vi "StopConnection.vi"(8 "ErrorIn":errorcluster, 11 "Reference":T1) -> (0 "ErrorOut":errorcluster)   [LabVIEW 2022 SP3]
uses:
  C:/Users/Robots/Documents/robocadSimLV/assemblies/LibraryForLabVIEW.dll
  assemblies/LibraryForLabVIEW.dll
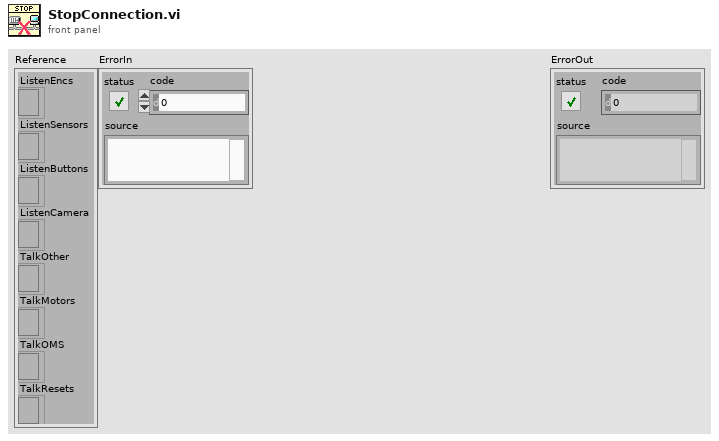
[diagram p1: front panel]
types:
  T1 = cluster{"ListenEncs":refnum<k24>, "ListenSensors":refnum<k24>, "ListenButtons":refnum<k24>, "ListenCamera":refnum<k24>, "TalkOther":refnum<k24>, "TalkMotors":refnum<k24>, "TalkOMS":refnum<k24>, "TalkResets":refnum<k24>}
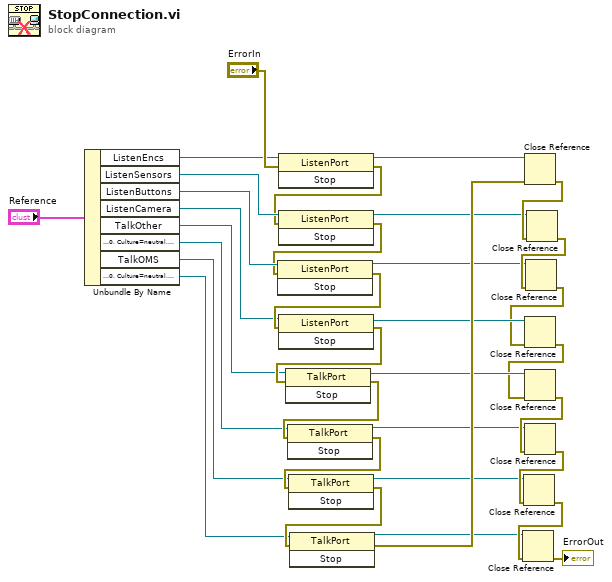
[diagram p0: block diagram]
diagram:
  n1 = Unbundle By Name("Reference") -> ("ListenEncs"=w32:refnum<k24>, "ListenSensors"=w31:refnum<k24>, "ListenButtons"=w29:refnum<k24>, "ListenCamera"=w26:refnum<k24>, "TalkOther"=w24:refnum<k24>, "TalkMotors"=w22:refnum<k24>, "TalkOMS"=w20:refnum<k24>, "TalkResets"=w18:refnum<k24>)
  n2 = invoke class="ListenPort" method="Stop"(reference=w32, error in="ErrorIn") -> (reference out=w17:refnum<k24>, error out=w30:errorcluster)  [unwired: 1 in, 1 out]
  n3 = invoke class="ListenPort" method="Stop"(reference=w31, error in=w30) -> (reference out=w14:refnum<k24>, error out=w28:errorcluster)  [unwired: 1 in, 1 out]
  n4 = invoke class="ListenPort" method="Stop"(reference=w29, error in=w28) -> (reference out=w12:refnum<k24>, error out=w27:errorcluster)  [unwired: 1 in, 1 out]
  n5 = invoke class="ListenPort" method="Stop"(reference=w26, error in=w27) -> (reference out=w11:refnum<k24>, error out=w25:errorcluster)  [unwired: 1 in, 1 out]
  n6 = invoke class="TalkPort" method="Stop"(reference=w24, error in=w25) -> (reference out=w9:refnum<k24>, error out=w23:errorcluster)  [unwired: 1 in, 1 out]
  n7 = invoke class="TalkPort" method="Stop"(reference=w22, error in=w23) -> (reference out=w6:refnum<k24>, error out=w21:errorcluster)  [unwired: 1 in, 1 out]
  n8 = invoke class="TalkPort" method="Stop"(reference=w20, error in=w21) -> (reference out=w4:refnum<k24>, error out=w19:errorcluster)  [unwired: 1 in, 1 out]
  n9 = invoke class="TalkPort" method="Stop"(reference=w18, error in=w19) -> (reference out=w2:refnum<k24>, error out=w16:errorcluster)  [unwired: 1 in, 1 out]
  n10 = Close Reference(reference=w17, error in (no error)=w16) -> (error out=w15:errorcluster)
  n11 = Close Reference(reference=w14, error in (no error)=w15) -> (error out=w13:errorcluster)
  n12 = Close Reference(reference=w12, error in (no error)=w13) -> (error out=w10:errorcluster)
  n13 = Close Reference(reference=w11, error in (no error)=w10) -> (error out=w8:errorcluster)
  n14 = Close Reference(reference=w9, error in (no error)=w8) -> (error out=w7:errorcluster)
  n15 = Close Reference(reference=w6, error in (no error)=w7) -> (error out=w5:errorcluster)
  n16 = Close Reference(reference=w4, error in (no error)=w5) -> (error out=w3:errorcluster)
  n17 = Close Reference(reference=w2, error in (no error)=w3) -> (error out=→"ErrorOut":errorcluster)
